vi "Config Type.vi"(11 "Start Log Command in":refnum<class "Start Log Command.lvclass">) -> (2 "Command Config Type":refnum<class "Command Config.lvclass">)   [LabVIEW 2020, in "VolatusSeq.lvlib" / "Start Log Command.lvclass"]
uses:
  Start Log Command.lvclass
  Start Log Command.lvclass/Start Log Command.ctl
  VolatusSeqConfig/Start Log Command Config/Start Log Command Config.lvclass
  C:/dev/lv20CE/relink/lv-volatus/VolatusSeqConfig/Command Config/Command Config.lvclass
  C:/dev/lv20CE/relink/lv-volatus/VolatusSeqConfig/Start Log Command Config/Start Log Command Config.lvclass
  VolatusSeqConfig/Command Config/Command Config.lvclass
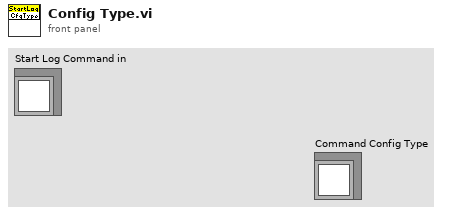
[diagram p1: front panel]
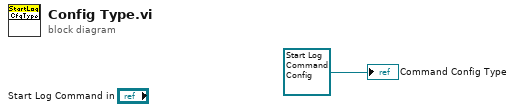
[diagram p0: block diagram]
diagram:
  "Command Config Type" <- refnum<class "Start Log Command Config.lvclass"> refnum ("VolatusSeqConfig.lvlib:Start Log Command Config.lvclass")
